vi "Load from JSON RTM.vi"(8 "error in (no error)":errorcluster, 11 "Node Ptr":u64 format="%.0x") -> (0 "error out":errorcluster)   [LabVIEW 2017, in "NI-SWITCH System Explorer.lvlib"]
uses:
  NI-SWITCH System Explorer.lvlib
  Scripting/SLSC Switch Scripting.lvlib
panel:
  in  "Tag":string
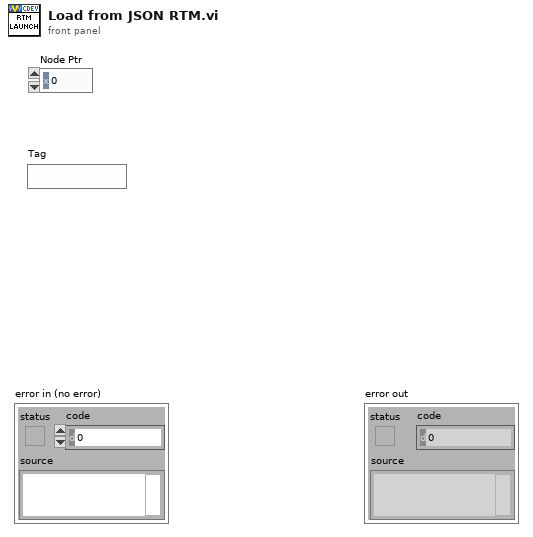
[diagram p1: front panel]
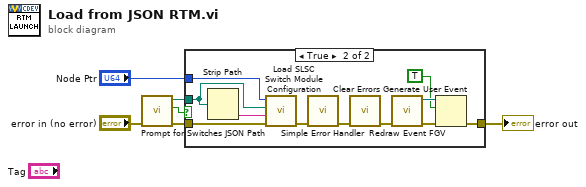
[diagram p0: block diagram]
diagram:
  n1 = call "Prompt for Switches JSON Path.vi"("error in (no error)"="error in (no error)") -> ("error out"=w3:errorcluster, "ok?"=w1:bool, "selected path"=w2:path)  [unwired: 8 in]
  n2 = case shown="True" w1 {
    tunnel: [w7 w15] -> w6
    tunnel: "Node Ptr" -> [_ w11]
    tunnel: w3 -> [w7 w10]
    tunnel: w2 -> [_ w8]
    frame False {
    }
    frame True {
      n3 = Strip Path(path=w8) -> (name=w9:string)  [unwired: 1 out]
      n4 = call "Load SLSC Switch Module Configuration.vi"("error in"=w10, "product name"=w9, "switches json file"=w8, "slsc switch custom device in"=w11) -> ("error out"=w14:errorcluster)  [unwired: 6 in, 1 out]
      n5 = call <vilib>:"Simple Error Handler.vi"("error in (no error)"=w14) -> ("error out"=w13:errorcluster)  [unwired: 4 in, 4 out]
      n6 = call <vilib>:"Clear Errors.vi"("error in (no error)"=w13) -> ("error out"=w12:errorcluster)  [unwired: 5 in, 1 out]
      n7 = call "Redraw Event FGV.vi"("error in (no error)"=w12) -> ("error out"=w18:errorcluster, "Redraw Event"=w17:refnum<user-event>)  [unwired: 9 in]
      n8 = Generate User Event(user event=w17, event data cluster=TRUE ("event data"), error in=w18) -> (error out=w15:errorcluster)  [unwired: 1 in, 1 out]
    }
  }
  "error out" <- w6
